vi "ProcessCalibrationData2.vi"(5 "Sensor Type":string, 9 "Use Div 5":bool, 10 "Fiducial 2":dbl[][](array[numeric]) format="%#_8g", 11 "Fiducial 1":dbl[][](array[numeric]) format="%#_8g") -> (2 "Avg Length":dbl format="%0.2f")   [LabVIEW 2019]
uses:
  <vilib>/Analysis/baseanly.llb/Mean (DBL).vi
  <vilib>/Analysis/NI_AALBase.lvlib
panel:
  # "Here a table of the co-ordinates for each interation of finding the fiducial can be found. Useful for debugging."
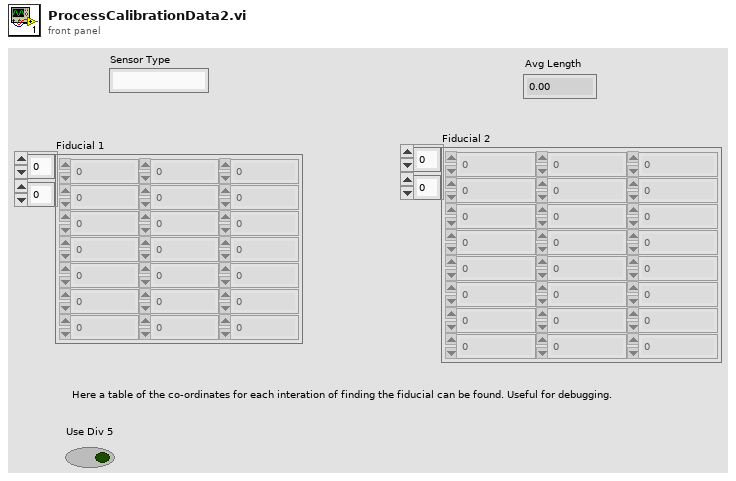
[diagram p1: front panel]
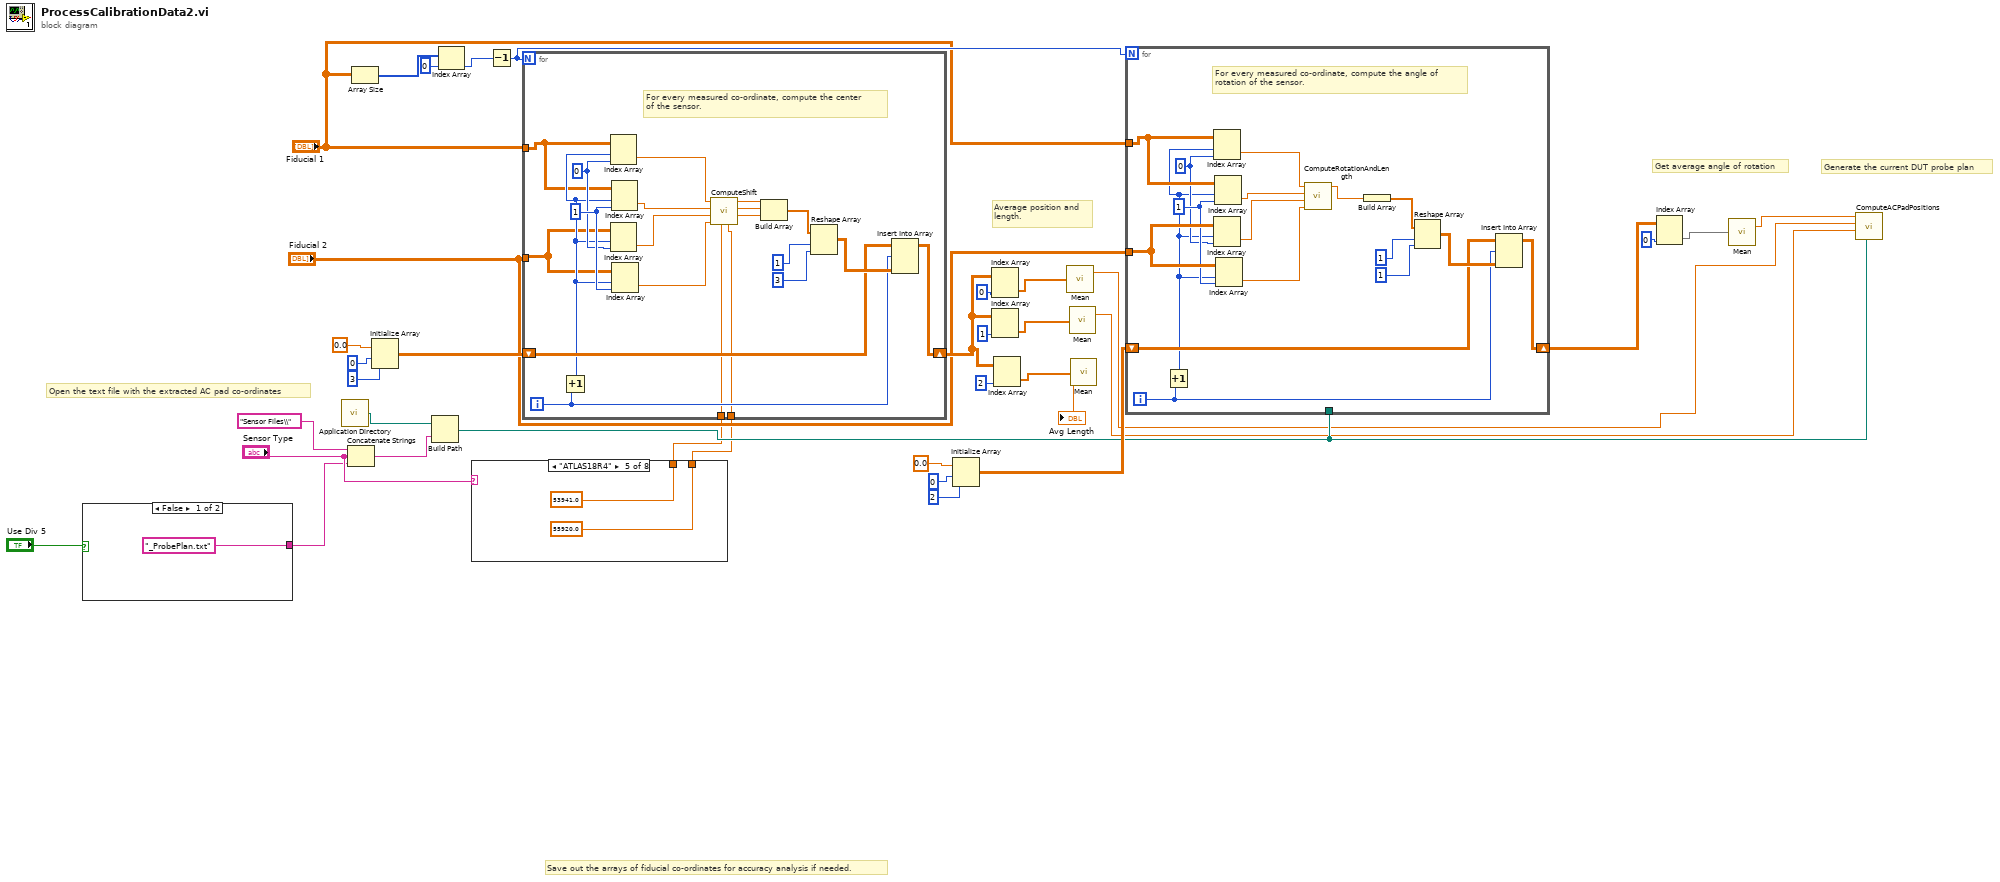
[diagram p0: block diagram]
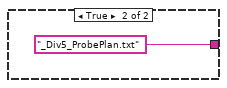
[diagram p2: hidden frame]
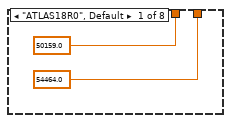
[diagram p3: hidden frame]
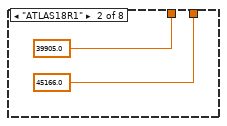
[diagram p4: hidden frame]
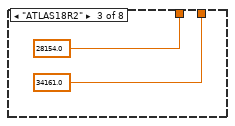
[diagram p5: hidden frame]
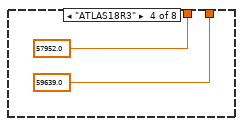
[diagram p6: hidden frame]
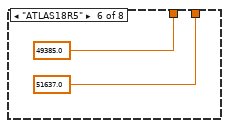
[diagram p7: hidden frame]
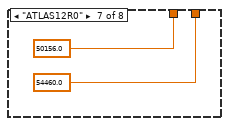
[diagram p8: hidden frame]
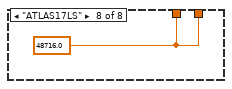
[diagram p9: hidden frame]
diagram:
  # "Generate the current DUT probe plan"
  # "Get average angle of rotation"
  # "Average position and\nlength."
  # "Save out the arrays of fiducial co-ordinates for accuracy analysis if needed."
  # "Open the text file with the extracted AC pad co-ordinates"
  n1 = case shown="False" "Use Div 5" {
    tunnel: ["_ProbePlan.txt" ("string") "_Div5_ProbePlan.txt" ("string")] -> w1
    frame False {
    }
    frame True {
    }
  }
  n2 = call <vilib>:"Application Directory.vi"() -> ("Application Directory"=w27:path)
  n3 = Concatenate Strings("Sensor Files\\" ("string"), "Sensor Type", w1) -> (w28:string)
  n4 = Array Size(array="Fiducial 1") -> (size(s)=w34:i32[])
  n5 = Initialize Array(0.0 ("element"), 0 ("dimension size"), 3 ("dimension size")) -> (w32:dbl[][])
  n6 = Build Path(base path=w27, name or relative path=w28) -> (appended path=w16:path)
  n7 = Index Array(array=w34, index=0) -> (element=w30:i32)
  n8 = case shown="\"ATLAS18R4\"" "Sensor Type" {
    tunnel: [50159.0 39905.0 28154.0 57952.0 53941.0 49385.0 50156.0 w54] -> w5
    tunnel: [54464.0 45166.0 34161.0 59639.0 55920.0 51637.0 54460.0 w54] -> w4
    frame "ATLAS18R0", Default {
    }
    frame "ATLAS18R1" {
    }
    frame "ATLAS18R2" {
    }
    frame "ATLAS18R3" {
    }
    frame "ATLAS18R4" {
    }
    frame "ATLAS18R5" {
    }
    frame "ATLAS12R0" {
    }
    frame "ATLAS17LS" {
      w54 = 48716.0
    }
  }
  n9 = Decrement(x=w30) -> (x-1=w17:i32)
  n10 = for {
    N: w17 -> [_]
    tunnel: "Fiducial 1" -> [w65]
    tunnel: "Fiducial 2" -> [w64]
    shift-right: [w69] -> w11
    shift-left: w32 -> [w68]
    tunnel: w5 -> [w56]
    tunnel: w4 -> [w55]
    i -> [w70]
    w75 = 1 ("disabled index (col)")
    w74 = 0 ("disabled index (col)")
    # "For every measured co-ordinate, compute the center\nof the sensor."
    n11 = Increment(x=w70) -> (x+1=w66:i32)
    n12 = Index Array(array=w65, index (row)=w66, index (col)=w74) -> (element=w60:dbl)
    n13 = Index Array(array=w64, index (row)=w66, index (col)=w74) -> (element=w62:dbl)
    n14 = Index Array(array=w65, index (row)=w66, index (col)=w75) -> (element=w61:dbl)
    n15 = Index Array(array=w64, index (row)=w66, index (col)=w75) -> (element=w63:dbl)
    n16 = call "ComputeShift.vi"("X1"=w60, "Y1"=w61, "X2"=w62, "Y2"=w63, "Dist Right"=w56, "Dist Left"=w55) -> ("XShift"=w59:dbl, "YShift"=w58:dbl, "Length"=w57:dbl)  [unwired: 2 in]
    n17 = Build Array(w59, w58, w57) -> (w72:dbl[])
    n18 = Reshape Array(w72, 1 ("dimension size"), 3 ("dimension size")) -> (w73:dbl[][])
    n19 = Insert Into Array(array=w68, index (row)=w70, new element=w73) -> (w69:dbl[][])  [unwired: 1 in]
  }
  n20 = Initialize Array(0.0 ("element"), 0 ("dimension size"), 2 ("dimension size")) -> (w18:dbl[][])
  n21 = Index Array(array=w11, index (col)=0 ("disabled index (col)")) -> (element=w26:dbl[])  [unwired: 1 in]
  n22 = Index Array(array=w11, index (col)=1 ("disabled index (col)")) -> (element=w25:dbl[])  [unwired: 1 in]
  n23 = Index Array(array=w11, index (col)=2 ("disabled index (col)")) -> (element=w9:dbl[])  [unwired: 1 in]
  n24 = call-poly <vilib>:"Mean.vi"("X"=w26) -> ("mean"=w14:dbl)  [unwired: 1 out]
  n25 = call-poly <vilib>:"Mean.vi"("X"=w25) -> ("mean"=w13:dbl)  [unwired: 1 out]
  n26 = call-poly <vilib>:"Mean.vi"("X"=w9) -> ("mean"=→"Avg Length":dbl)  [unwired: 1 out]
  n27 = for {
    N: w17 -> [_]
    tunnel: "Fiducial 1" -> [w92]
    tunnel: "Fiducial 2" -> [w91]
    shift-right: [w84] -> w12
    shift-left: w18 -> [w83]
    tunnel: w16 -> [_]
    i -> [w85]
    w90 = 1 ("disabled index (col)")
    w89 = 0 ("disabled index (col)")
    # "For every measured co-ordinate, compute the angle of \nrotation of the sensor."
    n28 = Increment(x=w85) -> (x+1=w81:i32)
    n29 = Index Array(array=w92, index (row)=w81, index (col)=w89) -> (element=w80:dbl)
    n30 = Index Array(array=w91, index (row)=w81, index (col)=w89) -> (element=w78:dbl)
    n31 = Index Array(array=w92, index (row)=w81, index (col)=w90) -> (element=w79:dbl)
    n32 = Index Array(array=w91, index (row)=w81, index (col)=w90) -> (element=w77:dbl)
    n33 = call "ComputeRotationAndLength.vi"("Y2"=w77, "X2"=w78, "Y1"=w79, "X1"=w80) -> ("Theta (Rad)"=w76:dbl)  [unwired: 7 in]
    n34 = Build Array(w76) -> (w87:dbl[])
    n35 = Reshape Array(w87, 1 ("dimension size"), 1 ("dimension size")) -> (w88:dbl[][])
    n36 = Insert Into Array(array=w83, index (row)=w85, new element=w88) -> (w84:dbl[][])  [unwired: 1 in]
  }
  n37 = Index Array(array=w12, index (col)=0 ("disabled index (col)")) -> (element=w22:dbl[])  [unwired: 1 in]
  n38 = call-poly <vilib>:"Mean.vi"("X"=w22) -> ("mean"=w15:dbl)  [unwired: 1 out]
  n39 = call "ComputeACPadPositions.vi"("Theta Calibration"=w15, "X cp"=w14, "Y cp"=w13, "Sensor Path"=w16) -> ()  [unwired: 7 in]
